vi "RWwrapper_enable.vi"(0 "Strings in":string[](array[string])=["C:\\CuspControl\\GPIB and Network\\Cusp\\u5wavefactoryname.txt", "6723"], 1 "Dubs in":dbl[](array[numeric])=[0.0]) -> ()   [LabVIEW 2018]
panel:
  in  "Enable":bool
  in  "Synth names file":path=path "C:/CuspControl/GPIB and Network/Cusp/u5wavefactoryname.txt"
  out "VISAsession":string="wavefactoryU5"
  in  "subvi":bool=TRUE
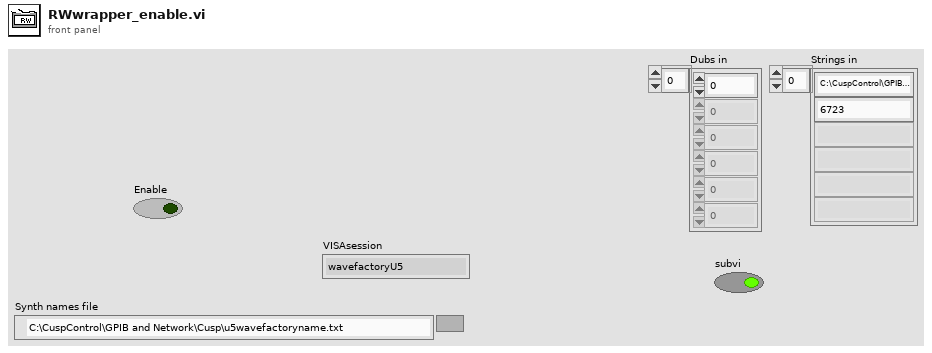
[diagram p1: front panel]
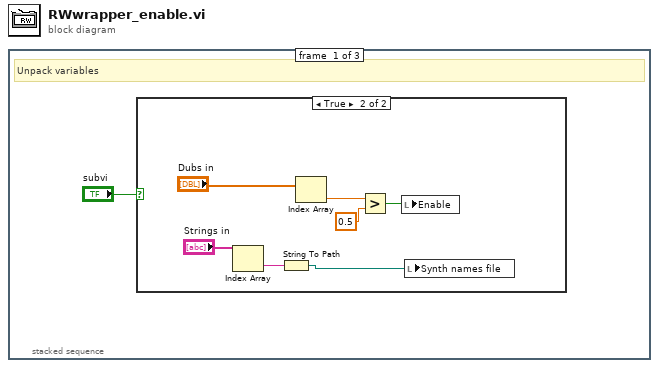
[diagram p0: block diagram]
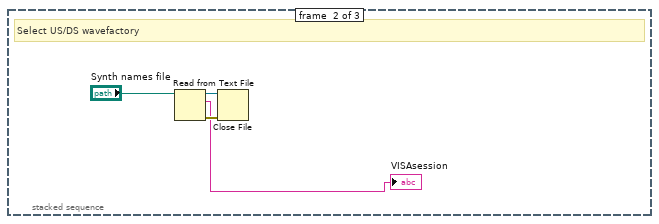
[diagram p3: hidden frame]
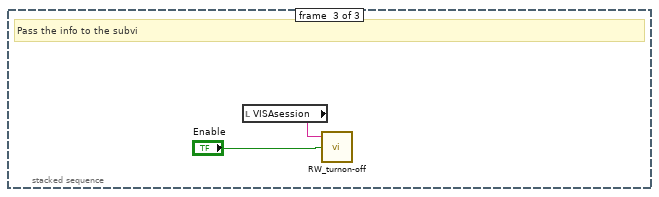
[diagram p4: hidden frame]
diagram:
  n1 = stacked-sequence {
    frame #0 {
      # "Unpack variables"
      n2 = case shown="True" "subvi" {
        frame False {
        }
        frame True {
          n3 = Index Array(array="Strings in") -> (element=w7:string)  [unwired: 1 in]
          n4 = String To Path(string=w7) -> (path=w6:path)
          n5 = Index Array(array="Dubs in") -> (element=w4:dbl)  [unwired: 1 in]
          n6 = Greater?(x=w4, y=0.5) -> (0:w2:bool)
          n7 = local write "Enable"(w2) -> ()
          n8 = local write "Synth names file"(w6) -> ()
        }
      }
    }
    frame #1 {
      # "Select US/DS wavefactory"
      n9 = Read from Text File(file (use dialog)="Synth names file") -> (refnum out=w10:refnum<file>, text=→"VISAsession":string, error out=w11:errorcluster)  [unwired: 3 in, 1 out]
      n10 = Close File(refnum=w10, error in=w11) -> ()  [unwired: 2 out]
    }
    frame #2 {
      # "Pass the info to the subvi"
      n11 = local read "VISAsession"() -> (w14:string)
      n12 = call "RW_turnon-off.vi"("On/Off"="Enable", "VISAsession"=w14) -> ()  [unwired: 2 in, 2 out]
    }
  }
